vi "Opponent.vi"(11 "Player":i32) -> (3 "Opponent":i32)   [LabVIEW 2017]
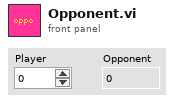
[diagram p1: front panel]
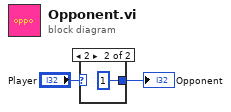
[diagram p0: block diagram]
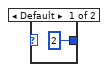
[diagram p2: hidden frame]
diagram:
  n1 = case shown="2" "Player" {
    tunnel: [2 ("Player") 1 ("Player")] -> w2
    frame Default {
    }
    frame 2 {
    }
  }
  "Opponent" <- w2
